vi "photo_encoder.vi"() -> ()   [LabVIEW 2014]
panel:
  out "Marks/second":dbl
  in  "Brightness of Mark":dbl
  in  "Photo Value(placeholder for sensor data)":dbl
  # "This VI recognizes significant increases in brightness as \"marks\" and outputs the number of marks detected in the last second.\nKnown issue:  Can only detect up to 1 mark per second.  Caused by \"wait\" block pausing the entire VI instead of just one section."
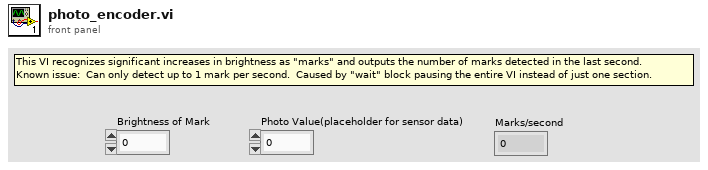
[diagram p1: front panel]
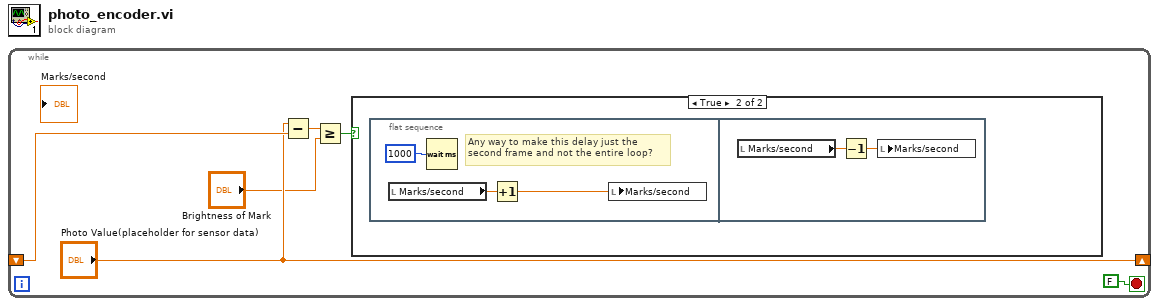
[diagram p0: block diagram]
diagram:
  n1 = while {
    shift-right: ["Photo Value(placeholder for sensor data)"] -> _
    shift-left: _ -> [w6]
    stop <- FALSE stop-if-true
    n2 = Subtract(x="Photo Value(placeholder for sensor data)", y=w6) -> (x-y=w4:dbl)
    n3 = Greater Or Equal?(x=w4, y="Brightness of Mark") -> (x >= y?=w2:bool)
    n4 = case shown="True" w2 {
      frame False {
      }
      frame True {
        n5 = flat-sequence {
          frame #0 {
            # "Any way to make this delay just the \nsecond frame and not the entire loop?"
            n6 = local read "Marks/second"() -> (w8:dbl)
            n7 = Wait (ms)(milliseconds to wait=u32 1000) -> ()  [unwired: 1 out]
            n8 = Increment(x=w8) -> (x+1=w7:dbl)
            n9 = local write "Marks/second"(w7) -> ()
          }
          frame #1 {
            n10 = local read "Marks/second"() -> (w11:dbl)
            n11 = Decrement(x=w11) -> (x-1=w10:dbl)
            n12 = local write "Marks/second"(w10) -> ()
          }
        }
      }
    }
  }
